vi "run.vi"(8 "error in (no error)":errorcluster, 11 "GenericImageAssembler in":refnum<class "GenericImageAssembler.lvclass">) -> (0 "error out":errorcluster, 3 "GenericImageAssembler out":refnum<class "GenericImageAssembler.lvclass">)   [LabVIEW 2010, in "GenericImageAssembler.lvclass"]
uses:
  GenericImageAssembler.lvclass
  common/classes/ErrorController/ErrorController/class_data.vi
  common/classes/ErrorController/ErrorController/ErrorController.lvclass
panel:
  # "Functionality not available..."
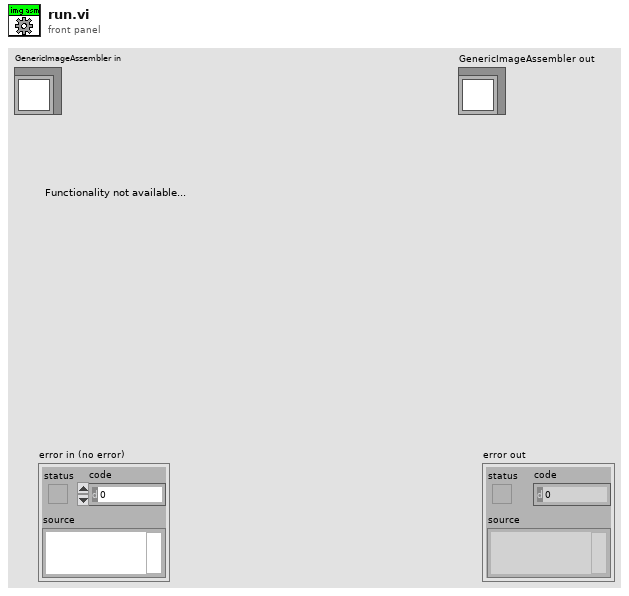
[diagram p1: front panel]
types:
  T1 = typedef "main_trigger_enum.ctl" = enum16{"NULL", "initialise", "terminate", "start", "stop", "change objective", "change experimentController", "change imagingMode", "save notebook", "started saving", "finished saving", "expCtr ready", "expCtr missing", "imgMd ready", "imgMd missing", "scanHd ready", "scanHd missing", "DAQ ready", "DAQ missing", "imgAsm ready", "imgAsm missing", "dataColl ready", "dataColl missing", "display ready", "display missing", "analysr ready", "analysr missing", "instrmnt ready", "instrmnt missing", "stimltr ready", "stimltr missing", "stage ready", "stage missing"}
  T2 = typedef "GenericToplevelComponent.lvclass/common_trigger_enum.ctl" = enum16{"NULL", "initialise", "terminate", "fetch command", "fetch data", "attach observer", "register as observer", "detach observer", "acknowledge", "start", "stop", "sweep started", "sweep finished", "experiment started", "experiment stopped"}
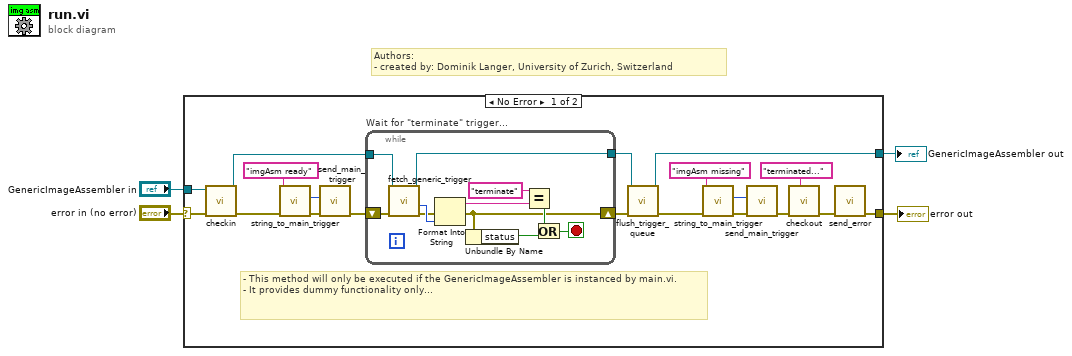
[diagram p0: block diagram]
diagram:
  # "Authors: \n- created by: Dominik Langer, University of Zurich, Switzerland"
  n1 = case shown="No Error" "error in (no error)" {
    selector: "error in (no error)" -> [w23 w36]
    tunnel: [w5 w36] -> w3
    tunnel: [w16 w35] -> w1
    tunnel: "GenericImageAssembler in" -> [w22 w35]
    frame No Error {
      # "- This method will only be executed if the GenericImageAssembler is instanced by main.vi.\n- It provides dummy functionality only..."
      n2 = call-dynamic "checkin.vi"("error in (no error)"=w23, "GenericImageAssembler in"=w22) -> ("error out"=w14:errorcluster, "GenericImageAssembler out"=w17:refnum<class "GenericImageAssembler.lvclass">)  [unwired: 8 in]
      n3 = call "string_to_main_trigger.vi"("error in (no error)"=w14, "trigger string"="imgAsm ready") -> ("error out"=w13:errorcluster, "main trigger"=w11:T1)  [unwired: 8 in]
      n4 = call "send_main_trigger.vi"("error in (no error)"=w13, "trigger"=w11) -> ("error out"=w20:errorcluster)  [unwired: 9 in]
      n5 = while "Wait for \"terminate\" trigger..." {
        shift-right: [w24] -> w19
        shift-left: w20 -> [w34]
        tunnel: w17 -> [w33]
        tunnel: [w29] -> w18
        stop <- w31 stop-if-true
        n6 = call-dynamic "fetch_generic_trigger.vi"("error in (no error)"=w34, "GenericToplevelComponent in"=w33) -> ("error out"=w25:errorcluster, "common trigger"=w28:T2, "GenericToplevelComponent out"=w29:refnum<class "GenericImageAssembler.lvclass">)  [unwired: 3 in, 4 out]
        n7 = Format Into String(error in=w25, w28) -> (resulting string=w27:string, error out=w24:errorcluster)  [unwired: 2 in]
        n8 = Unbundle By Name(w24) -> ("status"=w32:bool)
        n9 = Equal?(x="terminate", y=w27) -> (x = y?=w30:bool)
        n10 = Or(x=w30, y=w32) -> (x .or. y?=w31:bool)
      }
      n11 = call-dynamic "flush_trigger_queue.vi"("error in (no error)"=w19, "GenericToplevelComponent in"=w18) -> ("error out"=w10:errorcluster, "GenericToplevelComponent out"=w16:refnum<class "GenericImageAssembler.lvclass">)  [unwired: 8 in]
      n12 = call "string_to_main_trigger.vi"("error in (no error)"=w10, "trigger string"="imgAsm missing") -> ("error out"=w9:errorcluster, "main trigger"=w7:T1)  [unwired: 8 in]
      n13 = call "send_main_trigger.vi"("error in (no error)"=w9, "trigger"=w7) -> ("error out"=w21:errorcluster)  [unwired: 9 in]
      n14 = call "checkout.vi"("locked by?"="terminated...", "error in (no error)"=w21) -> ("error out"=w6:errorcluster)  [unwired: 8 in, 1 out]
      n15 = call "send_error.vi"("error in (no error)"=w6) -> ("error out"=w5:errorcluster)  [unwired: 10 in]
    }
    frame Error {
    }
  }
  "error out" <- w3
  "GenericImageAssembler out" <- w1
